vi "TestExec.Config, Get Station Module Info.vi"(8 "error in (no error)":errorcluster, 10 "Sta Module Path In":string="Applications\\Test Executive\\Modules\\TestExec.Example Station Module.vi", 11 "Sta Module Name In":string="Station Module") -> (0 "error out":errorcluster, 2 "Sta Module Path":string, 3 "Sta Module Name":string)   [LabVIEW 2018]
uses:
  <vilib>/Utility/config.llb/Read Key (String).vi
  <vilib>/Utility/config.llb/NI_LVConfig.lvlib
  <vilib>/KATE/Files/File Utils.lvlib
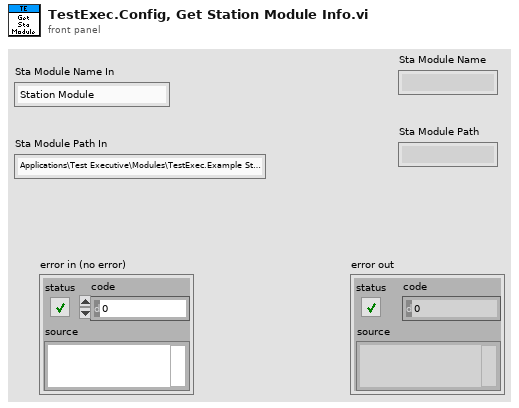
[diagram p1: front panel]
types:
  T1 = enum32{"invalid app kind", "Development System", "Run Time System", "Student Edition", "Embedded LabVIEW", "Evaluation", "Custom"}
  T2 = typedef "NI_LVConfig.lvlib/Config Data RefNum.ctl" = refnum<k1>
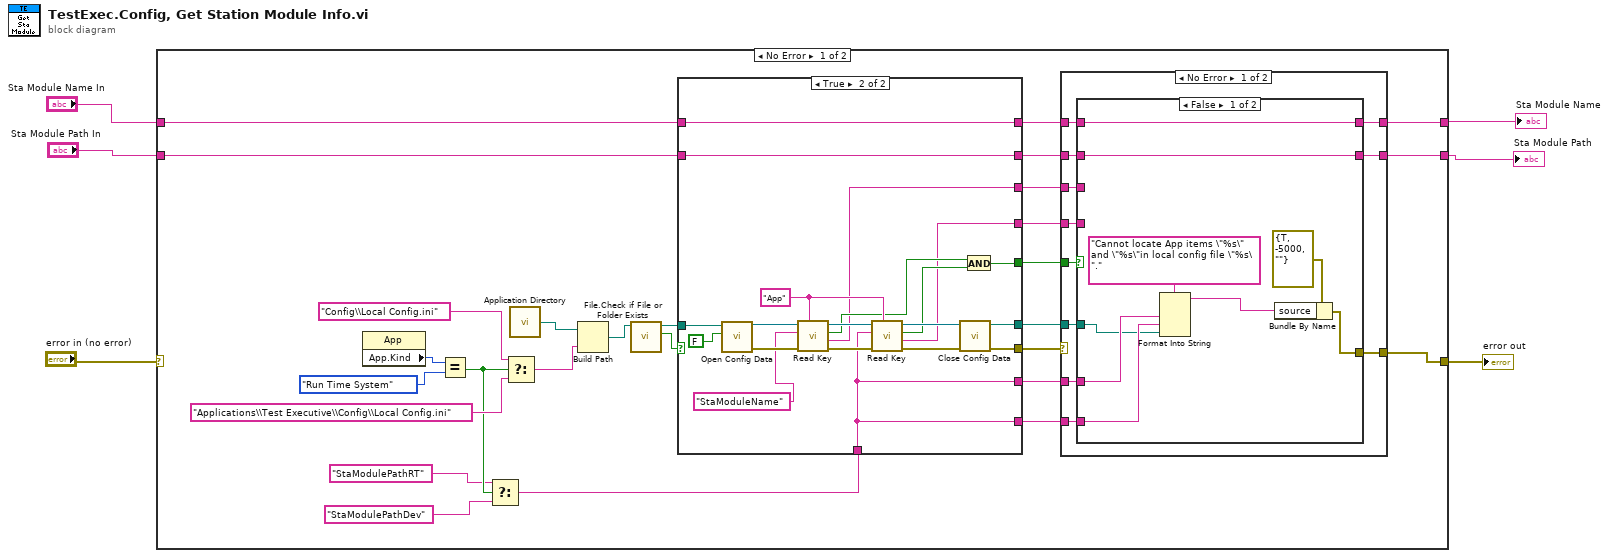
[diagram p0: block diagram]
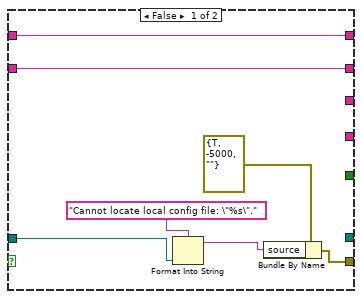
[diagram p4: hidden frame]
diagram:
  n1 = case shown="No Error" "error in (no error)" {
    selector: "error in (no error)" -> [_ w88]
    tunnel: [w12 w87] -> w2
    tunnel: [w10 w86] -> w1
    tunnel: [w17 w88] -> w5
    tunnel: "Sta Module Name In" -> [w14 w87]
    tunnel: "Sta Module Path In" -> [w13 w86]
    frame No Error {
      n2 = property class="App"() -> ("App.Kind"=w33:T1)  [unwired: 2 in, 2 out]
      n3 = Equal?(x=w33, y=T1."Run Time System" ("Application:Kind")) -> (x = y?=w27:bool)
      n4 = Select(t="StaModulePathRT" ("key"), s=w27, f="StaModulePathDev" ("key")) -> (s? t:f=w24:string)
      n5 = Select(t="Config\\Local Config.ini", s=w27, f="Applications\\Test Executive\\Config\\Local Config.ini") -> (s? t:f=w28:string)
      n6 = call <vilib>:"Application Directory.vi"() -> ("Application Directory"=w31:path)
      n7 = Build Path(base path=w31, name or relative path=w28) -> (appended path=w23:path)
      n8 = call <vilib>:"File.Check if File or Folder Exists.vi"("Path"=w23) -> ("Exists"=w21:bool, "Dup Path"=w22:path)  [unwired: 6 in, 3 out]
      n9 = case shown="True" w21 {
        tunnel: w24 -> [_ w67]
        tunnel: w22 -> [w62 w75]
        tunnel: [w60 w69] -> w11
        tunnel: [w59 w68] -> w9
        tunnel: [w61 w74] -> w16
        tunnel: [_ w73] -> w15
        tunnel: [_ w72] -> w20
        tunnel: [_ w67] -> w19
        tunnel: [_ w67] -> w18
        tunnel: w14 -> [w60 w69]
        tunnel: w13 -> [w59 w68]
        tunnel: [_ w71] -> w7
        tunnel: [_ w70] -> w8
        frame False {
          n10 = Format Into String(format string="Cannot locate local config file: \"%s\".", w62) -> (resulting string=w64:string)  [unwired: 2 in, 1 out]
          n11 = Bundle By Name(cluster=errorcluster {"status"=TRUE, "code"=-5000, "source"=""} ("error constant"), "source"=w64) -> (w61:errorcluster)
        }
        frame True {
          w78 = "App" ("section")
          n12 = call <vilib>:"Open Config Data.vi"("create file if necessary (T)"=FALSE, "configuration file path"=w75) -> ("error out"=w84:errorcluster, "refnum"=w85:T2)  [unwired: 7 in, 1 out]
          n13 = call-poly <vilib>:"Read Key.vi"("section"=w78, "error in (no error)"=w84, "key"="StaModuleName", "refnum"=w85) -> ("error out"=w81:errorcluster, "value"=w70:string, "found?"=w77:bool, "refnum out"=w82:T2)  [unwired: 4 in]
          n14 = call-poly <vilib>:"Read Key.vi"("section"=w78, "error in (no error)"=w81, "key"=w67, "refnum"=w82) -> ("error out"=w79:errorcluster, "value"=w71:string, "found?"=w76:bool, "refnum out"=w80:T2)  [unwired: 4 in]
          n15 = call <vilib>:"Close Config Data.vi"("error in (no error)"=w79, "refnum"=w80) -> ("error out"=w74:errorcluster, "file path"=w72:path)  [unwired: 8 in]
          n16 = And(x=w77, y=w76) -> (x .and. y?=w73:bool)
        }
      }
      n17 = case shown="No Error" w16 {
        selector: w16 -> [_ w58]
        tunnel: w20 -> [w42 _]
        tunnel: w19 -> [w44 _]
        tunnel: w18 -> [w43 _]
        tunnel: [w41 w58] -> w17
        tunnel: w15 -> [w40 _]
        tunnel: [w38 w57] -> w12
        tunnel: w11 -> [w39 w57]
        tunnel: [w37 w56] -> w10
        tunnel: w9 -> [w36 w56]
        tunnel: w8 -> [w35 _]
        tunnel: w7 -> [w34 _]
        frame No Error {
          n18 = case shown="False" w40 {
            tunnel: w44 -> [w51 _]
            tunnel: w43 -> [w50 _]
            tunnel: w42 -> [w49 _]
            tunnel: [w47 _] -> w41
            tunnel: w39 -> [w46 _]
            tunnel: [w46 w55] -> w38
            tunnel: [w45 w54] -> w37
            tunnel: w36 -> [w45 _]
            tunnel: w35 -> [_ w55]
            tunnel: w34 -> [_ w54]
            frame False {
              n19 = Format Into String(format string="Cannot locate App items \"%s\" and \"%s\"in local config file \"%s\".", w51, w50, w49) -> (resulting string=w48:string)  [unwired: 2 in, 1 out]
              n20 = Bundle By Name(cluster=errorcluster {"status"=TRUE, "code"=-5000, "source"=""} ("error constant"), "source"=w48) -> (w47:errorcluster)
            }
            frame True {
              # "OK"
            }
          }
        }
        frame Error {
        }
      }
    }
    frame Error {
    }
  }
  "Sta Module Path" <- w1
  "Sta Module Name" <- w2
  "error out" <- w5
